vi "OneShotButton.vi"(11 "Button In":bool) -> (3 "Boolean":bool)   [LabVIEW 2018]
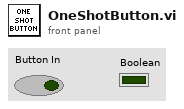
[diagram p1: front panel]
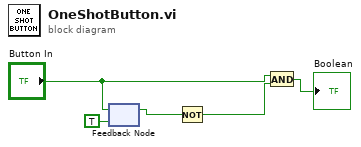
[diagram p0: block diagram]
diagram:
  n1 = feedback-in #1("Button In") -> ()
  n2 = feedback #1(TRUE ("Button In")) -> (w5:bool)
  n3 = Not(x=w5) -> (.not. x?=w3:bool)
  n4 = And(x="Button In", y=w3) -> (x .and. y?=→"Boolean":bool)
